vi "Build Specification_Get All Tags.vi"(0 "Build Spec reference in":refnum<vi>, 11 "error in(no error)":errorcluster) -> (4 "Build Spec reference out":refnum<vi>, 6 "Tag Names":string[](array[string]), 8 "Tag Values":variant[](array[variant]), 10 "Success?":bool, 15 "error out":errorcluster)   [LabVIEW 2019, in "ProjectBuilder.lvlib"]
doc: "List all build spec tags for the given build spec reference."
uses:
  ProjectBuilder.lvlib
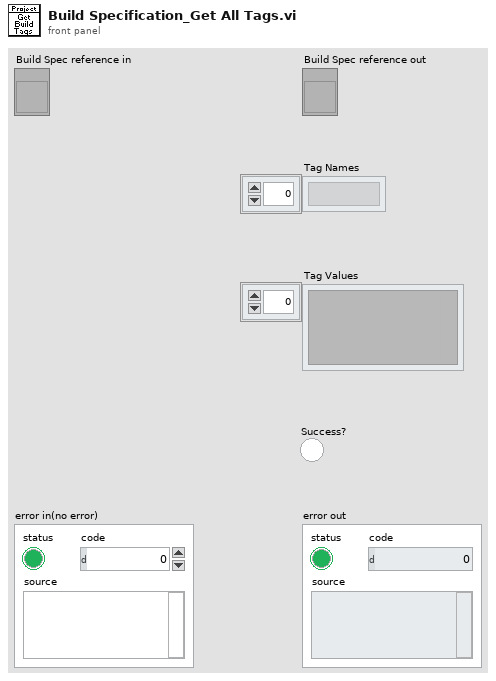
[diagram p1: front panel]
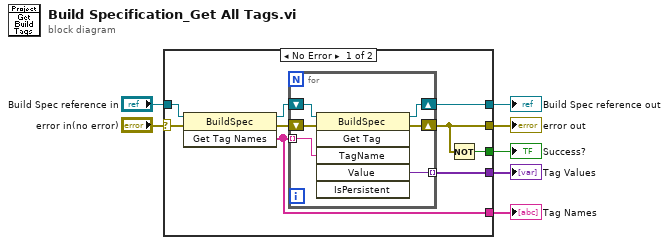
[diagram p0: block diagram]
diagram:
  n1 = case shown="No Error" "error in(no error)" {
    selector: "error in(no error)" -> [w13 w24]
    tunnel: [w11 w24] -> w6
    tunnel: "Build Spec reference in" -> [w16 w23]
    tunnel: [w10 _] -> w4
    tunnel: [w14 w23] -> w3
    tunnel: [w9 _] -> w2
    tunnel: [w8 _] -> w1
    frame No Error {
      n2 = invoke class="BuildSpec" method="Get Tag Names"(reference=w16, error in=w13) -> (reference out=w15:refnum<vi>, error out=w12:errorcluster, "Get Tag Names"=w8:string[])  [unwired: 1 in]
      n3 = for {
        tunnel: w8 -> [w21] mode=indexing
        shift-right: [w20] -> w14
        shift-left: w15 -> [w22]
        shift-right: [w18] -> w11
        shift-left: w12 -> [w19]
        tunnel: [w17] -> w9 mode=indexing
        n4 = invoke class="BuildSpec" method="Get Tag"(reference=w22, error in=w19, "TagName"=w21) -> (reference out=w20:refnum<vi>, error out=w18:errorcluster, "Value"=w17:variant)  [unwired: 3 in, 3 out]
      }
      n5 = Not(x=w11) -> (.not. x?=w10:bool)
    }
    frame Error {
    }
  }
  "error out" <- w6
  "Success?" <- w4
  "Build Spec reference out" <- w3
  "Tag Values" <- w2
  "Tag Names" <- w1
